vi "raster_scan_ground_shutter_new1.vi"() -> ()   [LabVIEW 2014] (continued)
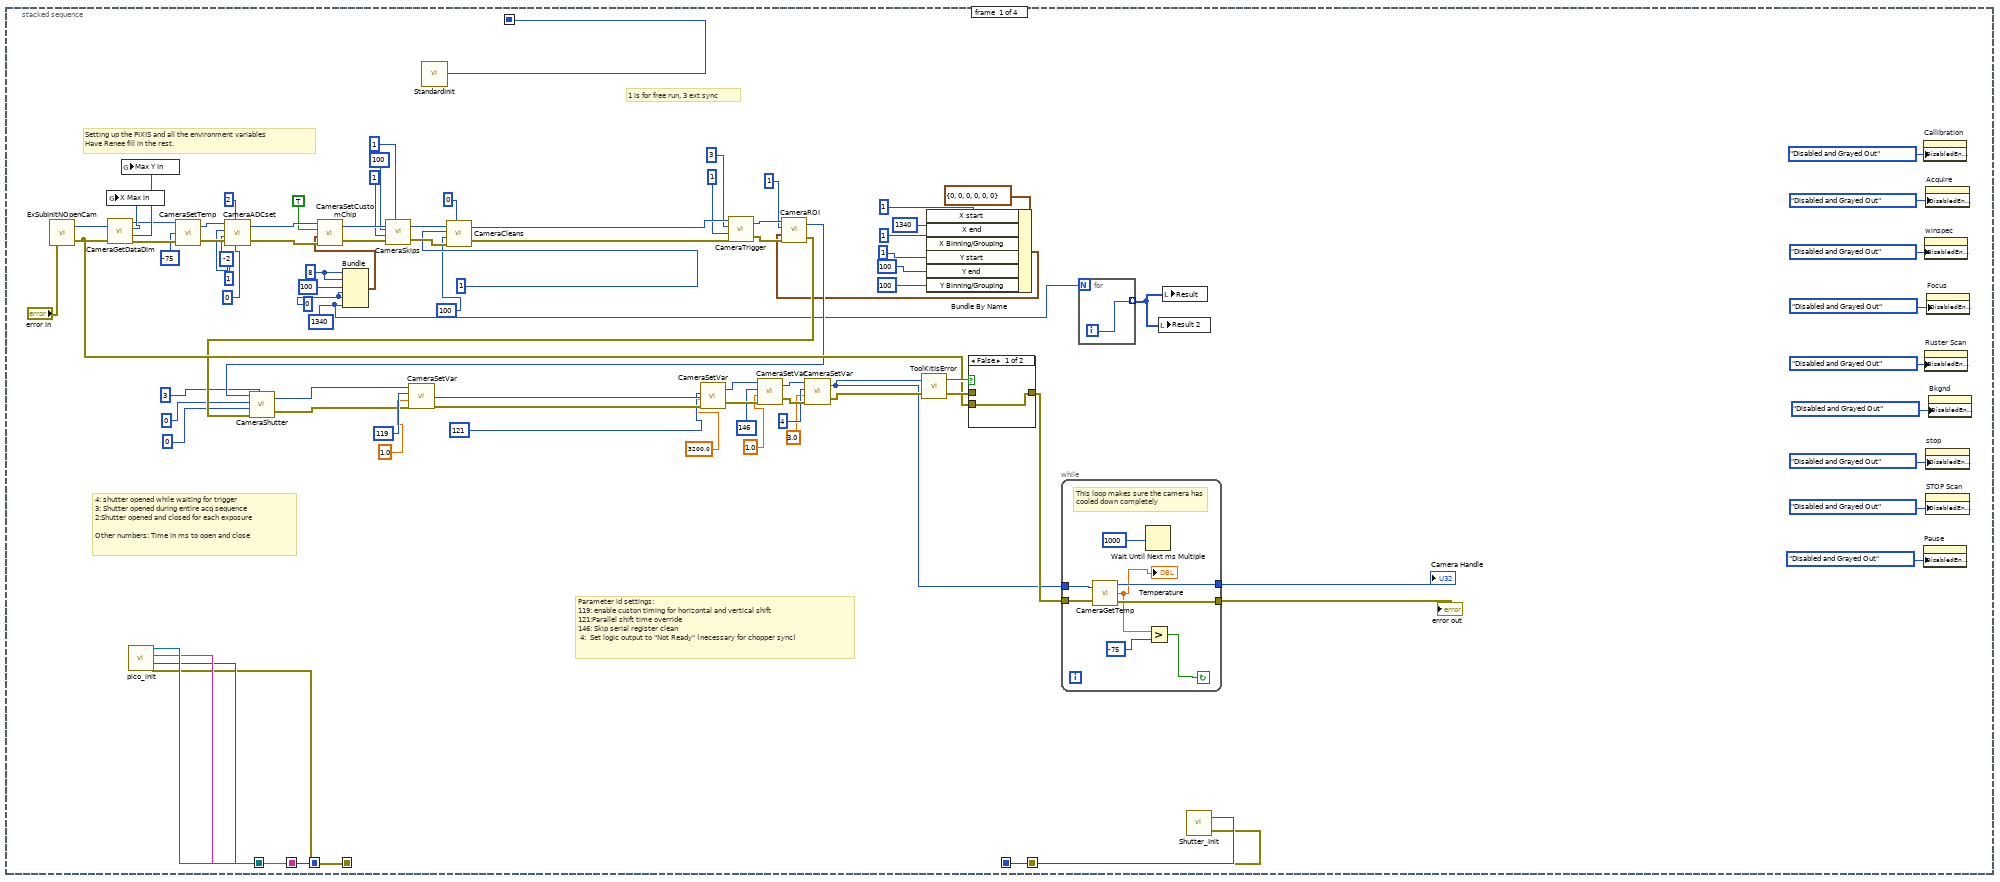
[diagram p2: hidden frame]
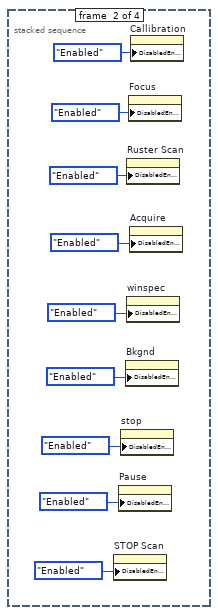
[diagram p4: hidden frame]
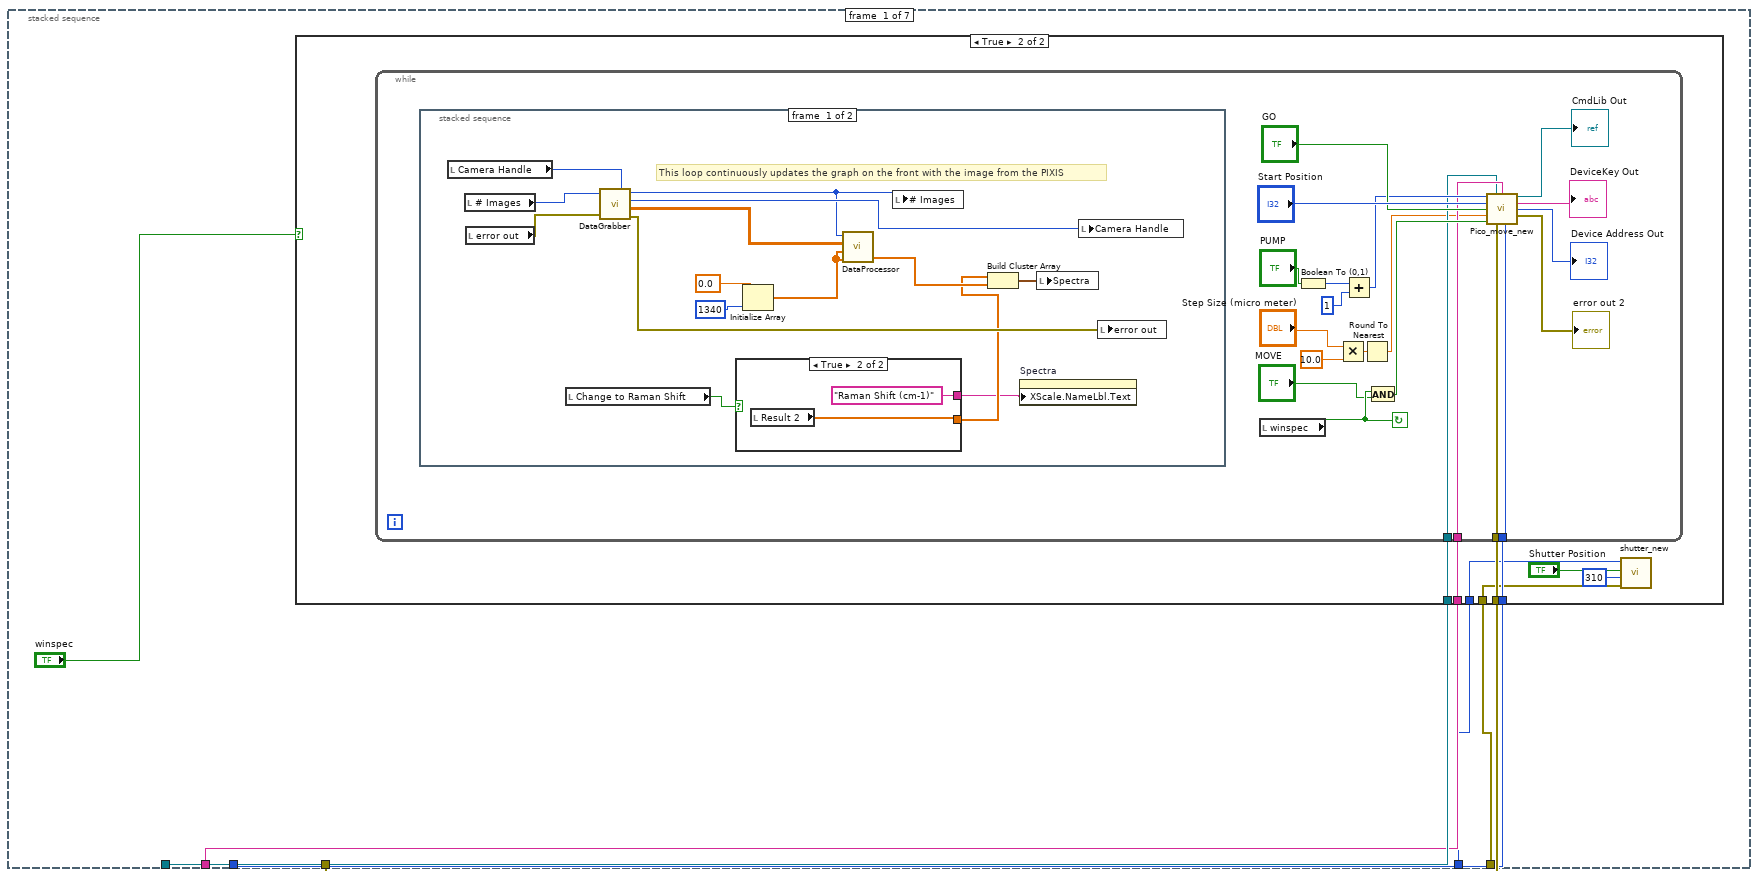
[diagram p5: hidden frame]
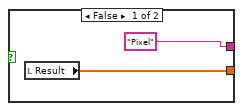
[diagram p7: hidden frame]
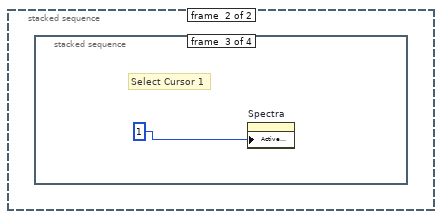
[diagram p8: hidden frame]
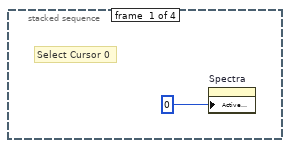
[diagram p9: hidden frame]
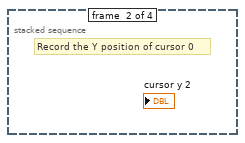
[diagram p10: hidden frame]
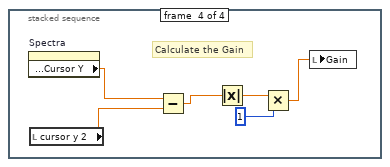
[diagram p11: hidden frame]
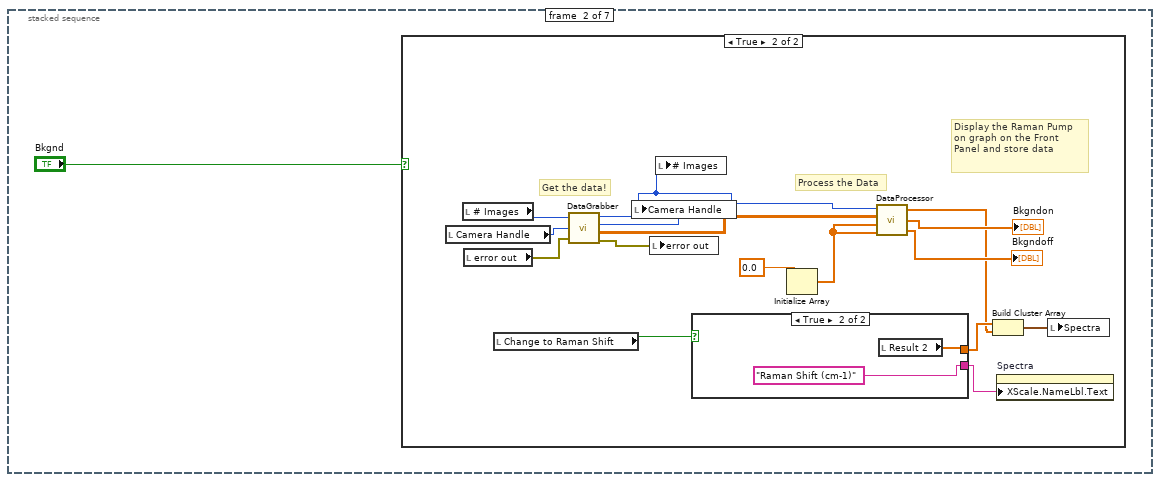
[diagram p12: hidden frame]
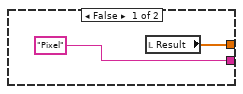
[diagram p14: hidden frame]
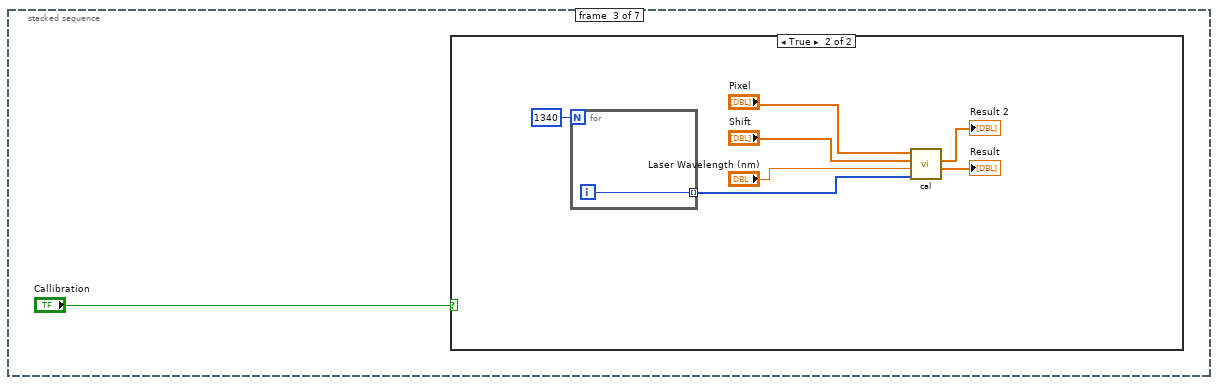
[diagram p15: hidden frame]
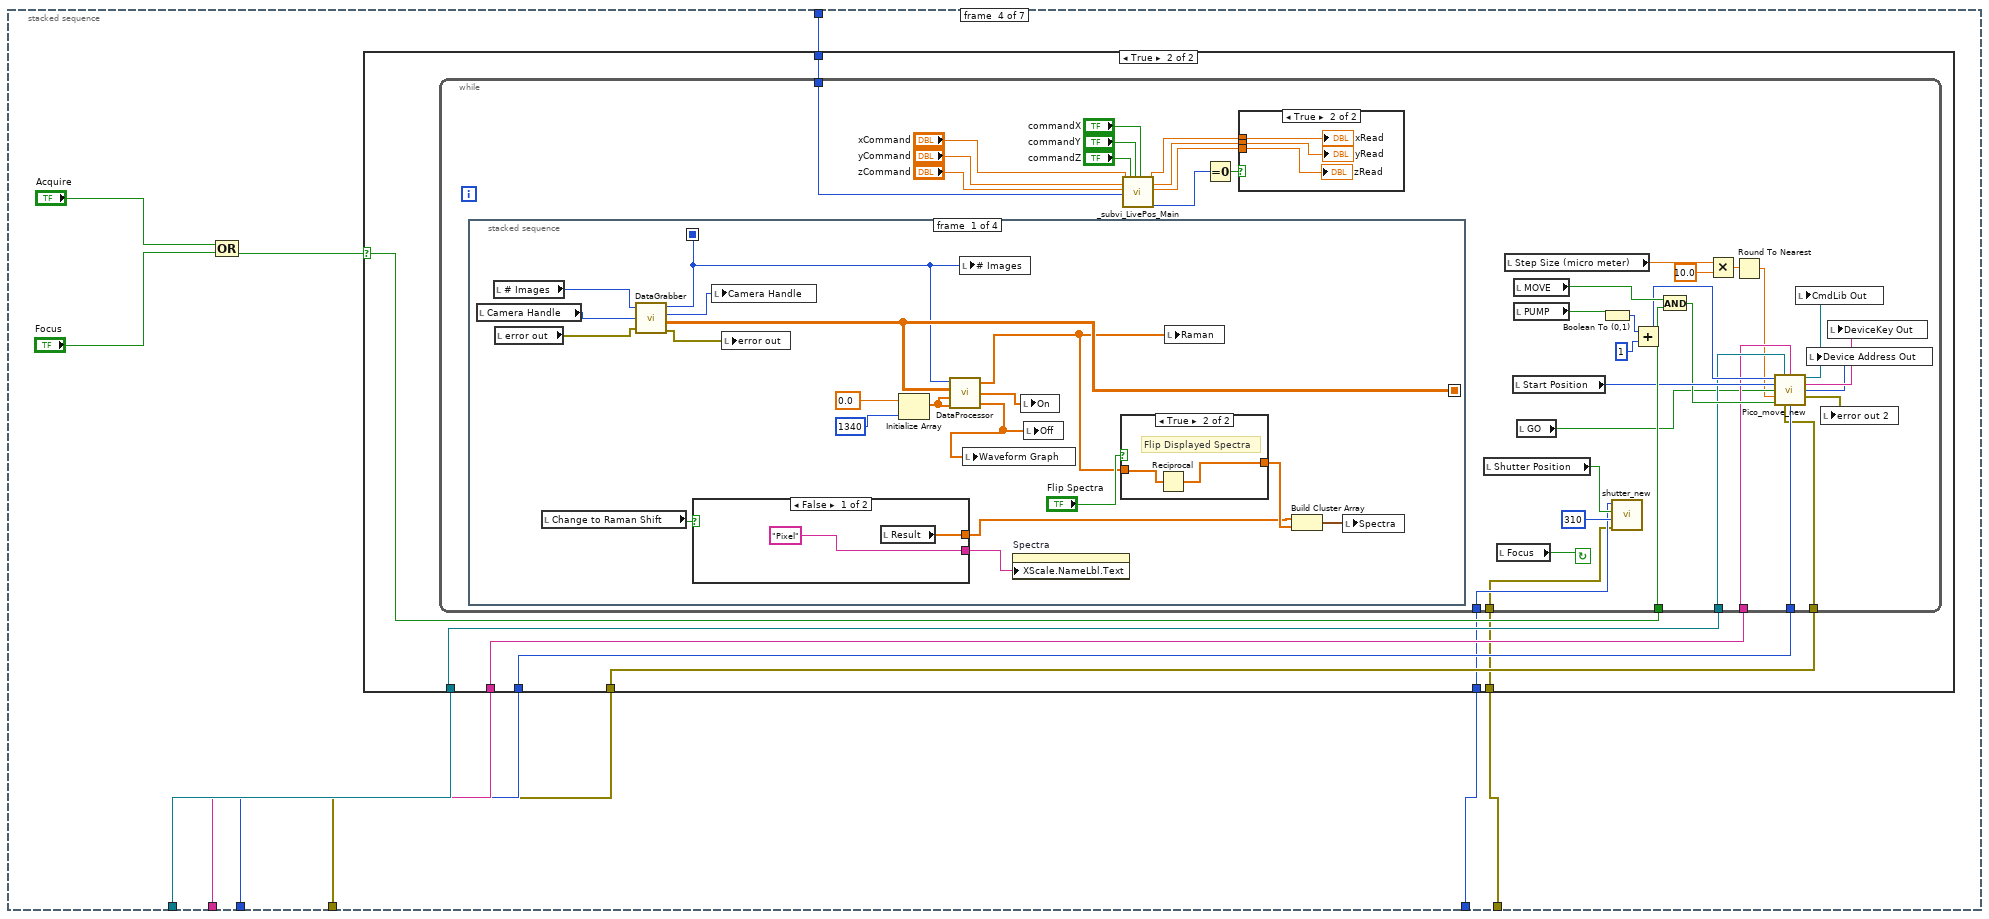
[diagram p17: hidden frame]
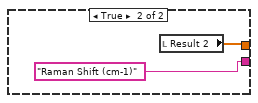
[diagram p20: hidden frame]
                      n435 = property on="Spectra" class="XYGraph (strict)"("XScale.NameLbl.Text"=w815) -> ()  [unwired: 2 in, 2 out]
                      n436 = local write "On"(w820) -> ()
                      n437 = local write "Off"(w821) -> ()
                      n438 = Not(x=w817) -> (.not. x?=w818:bool)
                      n439 = case shown="True" w818 {
                        tunnel: w814 -> [w834 w836]
                        tunnel: [w835 w836] -> w819
                        frame False {
                          n440 = Reciprocal(x=w834) -> (1/x=w835:dbl[])
                        }
                        frame True {
                        }
                      }
                      n441 = Build Cluster Array(w811, w819) -> (w816:cluster{dbl, dbl}[])
                      n442 = local write "Spectra"(w816) -> ()
                      n443 = local write "Raman"(w814) -> ()
                    }
                    frame #1 {
                      # "Here we save spectrum for each special point"
                      n444 = Increment(x=w838) -> (x+1=w837:i32)
                      n445 = local read "Filename"() -> (w841:string)
                      n446 = local read "Path"() -> (w843:string)
                      n447 = Format Into String(w837) -> (resulting string=w839:string)  [unwired: 3 in, 1 out]
                      n448 = Concatenate Strings(w843, "\\", w841, "_", w839) -> (w844:string)
                      n449 = local read "Off"() -> (w851:dbl[])
                      n450 = local read "On"() -> (w850:dbl[])
                      n451 = local read "Raman"() -> (w847:dbl[])
                      n452 = String To Path(string=w844) -> (path=w848:path)
                      n453 = Build Array(w847, w851, w850) -> (w849:dbl[][])
                      n454 = local write "File_name"(w844) -> ()
                      n455 = call-poly <vilib>:"Write To Spreadsheet File.vi"("transpose? (no:F)"=TRUE, "format (%.3f)"="%.7f", "2D data"=w849, "file path (dialog if empty)"=w848) -> ()  [unwired: 4 in, 1 out]
                    }
                    frame #2 {
                      # "Peak fitting and intergation"
                      n456 = local read "Raman"() -> (w858:dbl[])
                      n457 = property on="Spectra" class="XYGraph (strict)"("Active Cursor"=u32 1) -> ("Cursor.Cursor X"=w860:dbl)  [unwired: 2 in, 2 out]
                      n458 = local read "Enum"() -> (w855:enum16{"Lorantzian", "fano", "gaussian"})
                      n459 = property on="Spectra" class="XYGraph (strict)"("Active Cursor"=u32 0) -> ("Cursor.Cursor X"=w861:dbl)  [unwired: 2 in, 2 out]
                      n460 = call "fit_new.vi"("Cursor1 2"=w860, "Cursor1"=w861, "array 2"=w857, "array"=w858, "Enum"=w855, "Initial Parameters"="Fano initial Parameters 2") -> ("Intergrate"=w856:dbl, "Fit"=w852:dbl)  [unwired: 4 in]
                      n461 = local write "FIT"(w852) -> ()
                      n462 = local write "AREA"(w856) -> ()
                      n463 = Build Array (concatenate)(w853, w852) -> (w854:dbl[])
                      "Waveform Graph" <- w854
                    }
                  }
                }
              }
            }
          }
        }
      }
    }
    frame #3 {
      n464 = local read "DeviceKey Out"() -> (w866:string)
      n465 = local read "error out 2"() -> (w865:errorcluster)
      n466 = local read "CmdLib Out"() -> (w867:refnum<k24>)
      n467 = stacked-sequence {
        frame #0 {
          n468 = local read "Camera Handle"() -> (w868:u32)
          n469 = local read "error out"() -> (w869:errorcluster)
          n470 = call <userlib>:"CameraClose.vi"("error in"=w869, "Camera Handle"=w868) -> ("error out"=w871:errorcluster)
          n471 = call <userlib>:"UninitToolkit.vi"("error in"=w871) -> ("error out"=w870:errorcluster)
          n472 = local write "error out"(w870) -> ()
        }
      }
      n473 = call <instrlib>:"DeviceClose.vi"("error in (no error)"=w865, "DeviceKey In"=w866, "CmdLib In"=w867) -> ()  [unwired: 2 in, 3 out]
      n474 = dll-call lib="C:/Program Files/Mad City Labs/NanoDrive/Labview Examples/MADLib.dll" fn="MCL_ReleaseHandle"("handle"=w864) -> ()  [unwired: 5 in, 2 out]
    }
  }
